vi "FPGA Time to LabVIEW Time.vi"(1 "FPGA time (ns)":u64) -> (0 "LabVIEW time":timestamp)   [LabVIEW 2015, in "FPGA Timekeeper.lvlib"]
doc: "Converts FPGA Time into LabVIEW Time. Note that the FPGA Timekeeper keeps time in nanoseconds starting from January 1st, 1970."
uses:
  FPGA Timekeeper.lvlib
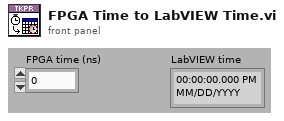
[diagram p1: front panel]
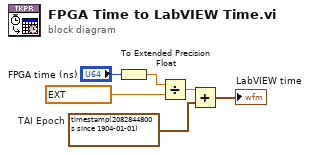
[diagram p0: block diagram]
diagram:
  w4 = timestamp(2082844800 s since 1904-01-01)  # TAI Epoch
  n1 = To Extended Precision Float(1:"FPGA time (ns)") -> (0:w1:ext)
  n2 = Divide(x=w1, y=ext 1000000000.0) -> (x/y=w5:ext)
  n3 = Add(x=w5, y=w4) -> (x+y=→"LabVIEW time":timestamp)
